vi "DAQ Init_Start_Switch.vi"() -> (1 "task out":refnum<k21>, 2 "error out":errorcluster)   [LabVIEW 2023]
uses:
  <vilib>/DAQmx/create/channels.llb/DAQmx Create Channel (DI-Digital Input).vi
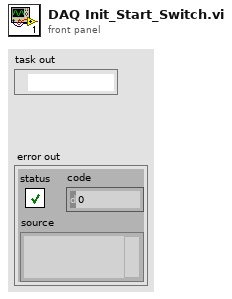
[diagram p1: front panel]
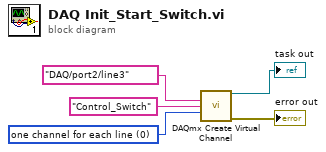
[diagram p0: block diagram]
diagram:
  w3 = 0 items=["one channel for each line", "one channel for all lines"] ("line grouping")
  n1 = call-poly <vilib>:"DAQmx Create Virtual Channel.vi"("lines"=tag "DAQ/port2/line3", "name to assign"="Control_Switch", "line grouping"=w3) -> ("task out"=→"task out":refnum<k21>, "error out"=→"error out":errorcluster)  [unwired: 11 in]
